vi "Get Size.vi"(8 "Error In":errorcluster, 11 "Display Manager In":refnum<class "Display Manager.lvclass">) -> (0 "Error Out":errorcluster, 2 "Size":T1, 3 "Display Manager Out":refnum<class "Display Manager.lvclass">)   [LabVIEW 2021, in "Display Manager.lvclass"]
uses:
  Display Manager.lvclass
  Display Utilities/Public/Controls/2D Dimensions.ctl
  Display Manager.lvclass/Display Manager.ctl
  Display Utilities/Display Utilities.lvlib
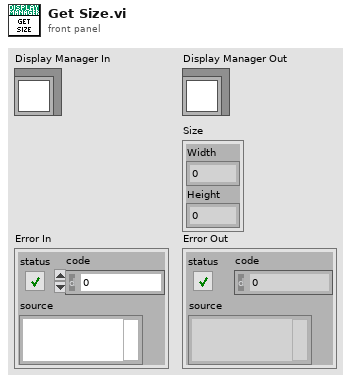
[diagram p1: front panel]
types:
  T1 = typedef "Display Utilities.lvlib/2D Dimensions.ctl" = cluster{"Width":i32, "Height":i32}
  T2 = typedef "Display Manager.lvclass/Data.ctl" = cluster{"Size":T1, "Display Elements":refnum<class "Display Element.lvclass">[], "Frame":u32[][]}
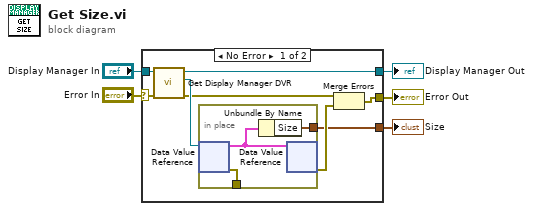
[diagram p0: block diagram]
diagram:
  n1 = case shown="No Error" "Error In" {
    selector: "Error In" -> [w9 w17]
    tunnel: [w11 w17] -> w4
    tunnel: [w8 w18] -> w3
    tunnel: "Display Manager In" -> [w10 w18]
    tunnel: [w12 _] -> w1
    frame No Error {
      n2 = call "Get Display Manager DVR.vi"("Error In"=w9, "Display Manager In"=w10) -> ("Error Out"=w6:errorcluster, "DVR"=w7:refnum<data-value>, "Display Manager Out"=w8:refnum<class "Display Manager.lvclass">)  [unwired: 7 in]
      n3 = in-place {
        in-place-border: [w14] -> w12
        in-place-border: [w16] -> _
        n4 = in-place-dvr #1(w7) -> (w15:T2, w16:errorcluster)
        n5 = Unbundle By Name(w15) -> ("Size"=w14:T1)
        n6 = in-place-dvr #1(w15) -> (w13:errorcluster)  [unwired: 1 out]
      }
      n7 = Merge Errors(w6, w13) -> (w11:errorcluster)
    }
    frame Error {
    }
  }
  "Error Out" <- w4
  "Display Manager Out" <- w3
  "Size" <- w1
